vi "INI Read Str.vi"(7 "Section Str":string="Params", 8 "error IN":errorcluster, 10 "Key Str":string, 11 "configuration file path":path=path "D:/3D FIB-SEM Files/FeissTEST.ini") -> (0 "error out":errorcluster, 2 "Str Out":string, 3 "file path Out":path)   [LabVIEW 2018]
uses:
  <vilib>/Utility/config.llb/Read Key (String).vi
  <vilib>/Utility/config.llb/NI_LVConfig.lvlib
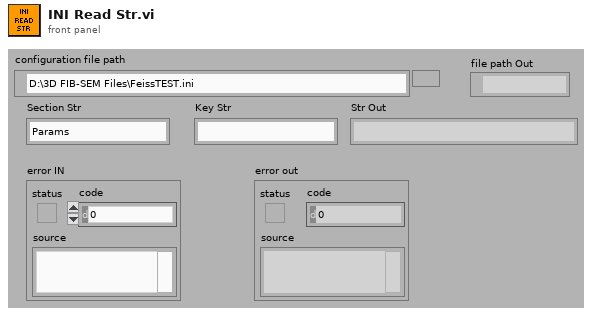
[diagram p1: front panel]
types:
  T1 = typedef "NI_LVConfig.lvlib/Config Data RefNum.ctl" = refnum<k1>
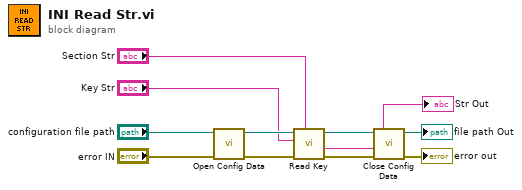
[diagram p0: block diagram]
diagram:
  n1 = call <vilib>:"Open Config Data.vi"("error in (no error)"="error IN", "configuration file path"="configuration file path") -> ("error out"=w7:errorcluster, "refnum"=w9:T1)  [unwired: 7 in, 1 out]
  n2 = call-poly <vilib>:"Read Key.vi"("section"="Section Str", "error in (no error)"=w7, "key"="Key Str", "refnum"=w9) -> ("error out"=w6:errorcluster, "value"=→"Str Out":string, "refnum out"=w8:T1)  [unwired: 4 in, 1 out]
  n3 = call <vilib>:"Close Config Data.vi"("error in (no error)"=w6, "refnum"=w8) -> ("error out"=→"error out":errorcluster, "file path"=→"file path Out":path)  [unwired: 8 in]
